vi "ApplyGain.vi"(7 "reset":bool, 8 "input valid":bool, 10 "gain":T1={"gain I"=1.0, "gain Q"=1.0}, 11 "data in":T2[](array[typedef])=[{"I"=0.0, "Q"=0.0, "overflow"=FALSE}, {"I"=0.0, "Q"=0.0, "overflow"=FALSE}, {"I"=0.0, "Q"=0.0, "overflow"=FALSE}, {"I"=0.0, "Q"=0.0, "overflow"=FALSE}]) -> (0 "output valid":bool, 3 "data out":T2[](array[typedef]))   [LabVIEW 2025]
uses:
  <instrlib>/_niInstr/DSP/v1/FPGA/niInstr DSP v1 FPGA.lvlib
  <instrlib>/_niInstr/DSP/v1/Shared/Public/IQ Data.ctl
  <instrlib>/_niInstr/DSP/v1/Shared/niInstr DSP v1 Shared.lvlib
  <instrlib>/_niInstr/DSP/v1/Shared/Public/IQ Gain.ctl
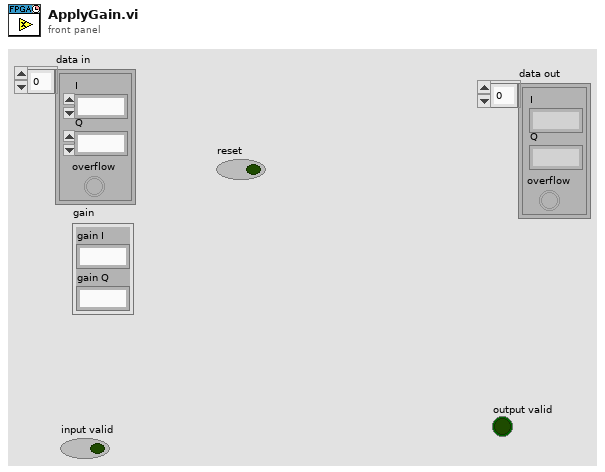
[diagram p1: front panel]
types:
  T1 = typedef "niInstr DSP v1 Shared.lvlib/IQ Gain.ctl" = cluster{"gain I":fxp<+/-,24,3>, "gain Q":fxp<+/-,24,3>}
  T2 = typedef "niInstr DSP v1 Shared.lvlib/IQ Data.ctl" = cluster{"I":fxp<+/-,18,1>, "Q":fxp<+/-,18,1>, "overflow":bool}
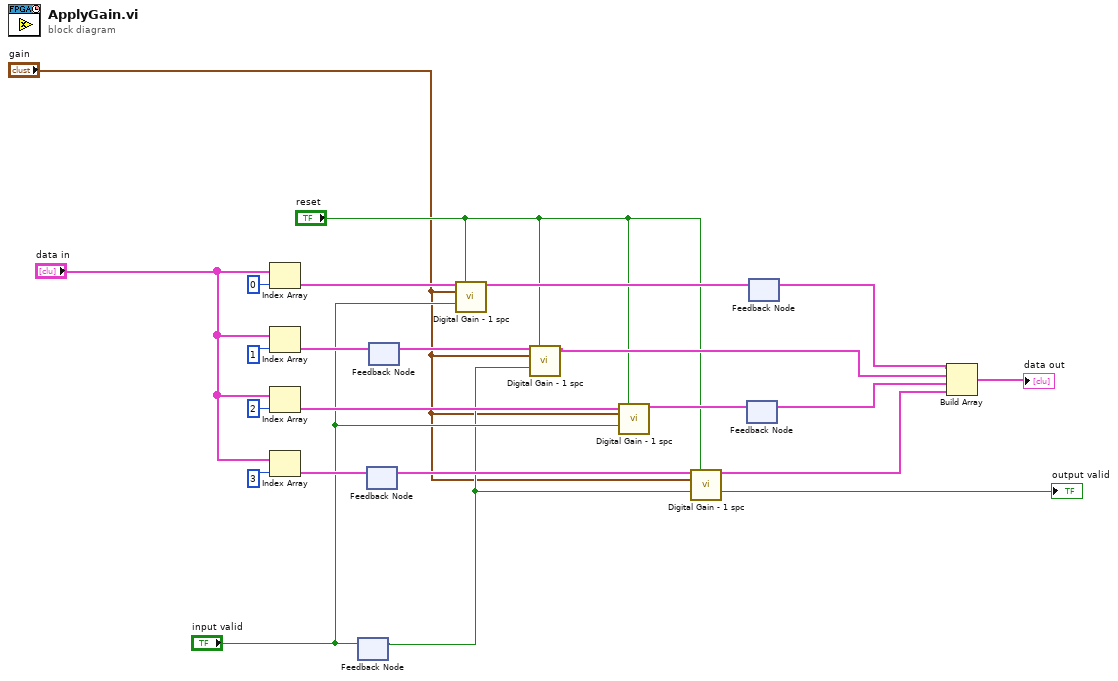
[diagram p0: block diagram]
diagram:
  n1 = Index Array(array="data in", index=0) -> (element=w13:T2)
  n2 = Index Array(array="data in", index=1) -> (element=w18:T2)
  n3 = Index Array(array="data in", index=2) -> (element=w9:T2)
  n4 = Index Array(array="data in", index=3) -> (element=w17:T2)
  n5 = feedback #1() -> (w3:bool)  [unwired: 1 in]
  n6 = feedback-in #1("input valid") -> ()
  n7 = feedback #2() -> (w6:T2)  [unwired: 1 in]
  n8 = feedback-in #2(w17) -> ()
  n9 = feedback #3() -> (w11:T2)  [unwired: 1 in]
  n10 = feedback-in #3(w18) -> ()
  n11 = call <instrlib>:"Digital Gain - 1 spc.vi"("data in"=w13, "reset"="reset", "gain"="gain", "input valid"="input valid") -> ("data out"=w12:T2)  [unwired: 8 in, 3 out]
  n12 = call <instrlib>:"Digital Gain - 1 spc.vi"("data in"=w11, "reset"="reset", "gain"="gain", "input valid"=w3) -> ("data out"=w10:T2)  [unwired: 8 in, 3 out]
  n13 = call <instrlib>:"Digital Gain - 1 spc.vi"("data in"=w9, "reset"="reset", "gain"="gain", "input valid"="input valid") -> ("data out"=w8:T2)  [unwired: 8 in, 3 out]
  n14 = call <instrlib>:"Digital Gain - 1 spc.vi"("data in"=w6, "reset"="reset", "gain"="gain", "input valid"=w3) -> ("data out"=w5:T2, "output valid"=→"output valid":bool)  [unwired: 8 in, 2 out]
  n15 = feedback #4() -> (w15:T2)  [unwired: 1 in]
  n16 = feedback-in #4(w8) -> ()
  n17 = feedback #5() -> (w16:T2)  [unwired: 1 in]
  n18 = feedback-in #5(w12) -> ()
  n19 = Build Array(w16, w10, w15, w5) -> (→"data out":T2[])
